vi "GetMaxVeloc.vi"(11 "CurrenMeters":cluster{"Array":timestamp[], "Array":dbl[]}[](array[cluster])) -> (2 "TimeStamps":timestamp[](array[timestamp]), 3 "MaxVelocs":dbl[](array[numeric]))   [LabVIEW 2016]
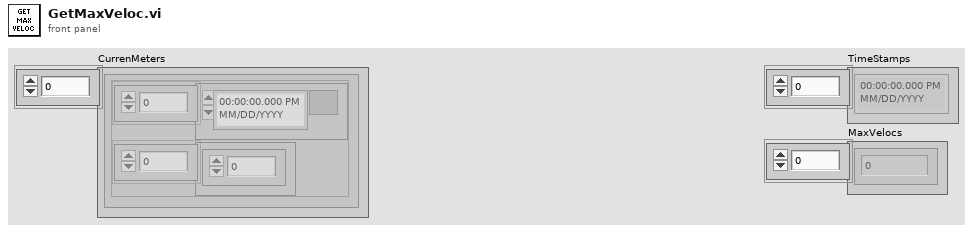
[diagram p1: front panel]
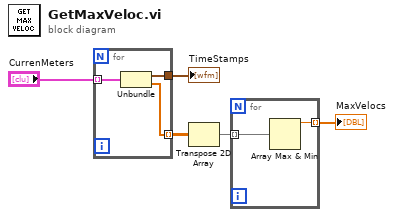
[diagram p0: block diagram]
diagram:
  n1 = for {
    tunnel: "CurrenMeters" -> [w8] mode=indexing
    tunnel: [w7] -> w2
    tunnel: [w6] -> w4 mode=indexing
    n2 = Unbundle(w8) -> ("Array"=w7:timestamp[], "Array"=w6:dbl[])
  }
  "TimeStamps" <- w2
  n3 = Transpose 2D Array(2D array=w4) -> (transposed array=w3:dbl[][])
  n4 = for {
    tunnel: w3 -> [w10] mode=indexing
    tunnel: [w9] -> w1 mode=indexing
    n5 = Array Max & Min(array=w10) -> (max value=w9:dbl)  [unwired: 3 out]
  }
  "MaxVelocs" <- w1
